vi "Ctor.vi"(7 "Platforms":refnum<class "PlatformManager.lvclass">, 8 "error in (no error)":errorcluster, 10 "Resource":refnum<class "Resource.lvclass">, 11 "Platform":refnum<class "Platform.lvclass">) -> (0 "error out":errorcluster, 3 "Device out":refnum<class "Device.lvclass">)   [LabVIEW 2020, in "PicoG-App.lvlib" / "Device.lvclass"]
uses:
  Device.lvclass
  Builds/picoG/ppl/PicoG-Core.lvlibp/PicoG-Processor/PicoG-Core/Platform/Platform.lvclass
  Builds/picoG/ppl/PicoG-Core.lvlibp/PicoG-Processor/PicoG-Core/Resource/Resource.lvclass
  Builds/picoG/ppl/PicoG-Core.lvlibp/PicoG-Processor/PicoG-Core/PlatformManager/PlatformManager.lvclass
  Resource Ref.ctl
  Ref Data.ctl
  Device Key.ctl
  Device.lvclass/Device.ctl
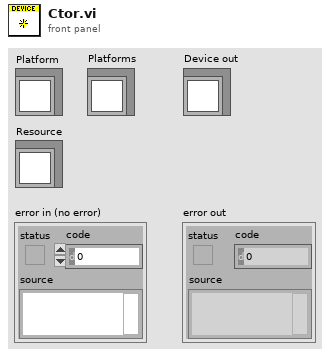
[diagram p1: front panel]
types:
  T1 = typedef "PicoG-App.lvlib/Device.lvclass/Ref Data.ctl" = cluster{"Alias":string, "Version":string, "Build":timestamp, "Key":T2}
  T2 = typedef "PicoG-App.lvlib/Device.lvclass/Device Key.ctl" = cluster{"Platform":string, "Board":string, "ID":string}
  T3 = typedef "PicoG-App.lvlib/Device.lvclass/Resource Ref.ctl" = cluster{"Resource":refnum<class "Resource.lvclass">, "Open":bool, "At Prompt":bool, "Running":bool}
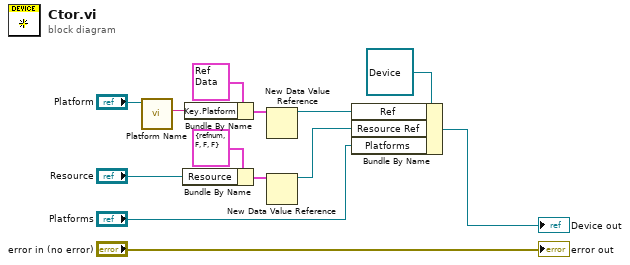
[diagram p0: block diagram]
diagram:
  n1 = call-dynamic "Platform Name.vi"("DeployTarget in"="Platform") -> ("Platform Name"=w4:string)  [unwired: 8 in, 2 out]
  n2 = Bundle By Name(cluster=T3 {"Resource"=refnum, "Open"=FALSE, "At Prompt"=FALSE, "Running"=FALSE} ("Resource Ref"), "Resource"="Resource") -> (w7:T3)
  n3 = Bundle By Name(cluster=T1 {"Alias"="", "Version"="", "Build"=timestamp(0 s since 1904-01-01), "Key"={"Platform"="", "Board"="", "ID"=""}} ("Ref Data"), "Key.Platform"=w4) -> (w3:T1)
  n4 = New Data Value Reference(data value=w3) -> (data value reference=w2:refnum<data-value>)  [unwired: 1 in, 1 out]
  n5 = New Data Value Reference(data value=w7) -> (data value reference=w6:refnum<data-value>)  [unwired: 1 in, 1 out]
  n6 = Bundle By Name(cluster=refnum<class "Device.lvclass"> refnum ("Device in"), "Ref"=w2, "Resource Ref"=w6, "Platforms"="Platforms") -> (→"Device out":refnum<class "Device.lvclass">)
  "error out" <- "error in (no error)"
